vi "Actividad_01_Completa.vi"() -> ()   [LabVIEW 2025]
uses:
  <vilib>/Instr/_visa.llb/VISA Configure Serial Port (Instr).vi
panel:
  out "Contador":i32(knob) scale=-10000.0..10000.0
  out "Temperatura":dbl(slide) scale=0.0..100.0
  out "substring 2":string
  out "substring":string
  out "Temperatura buena":dbl
  out "Contador motor":i32
  in  "stop":bool
  in  "VISA resource name":refnum<visa-resource-name>
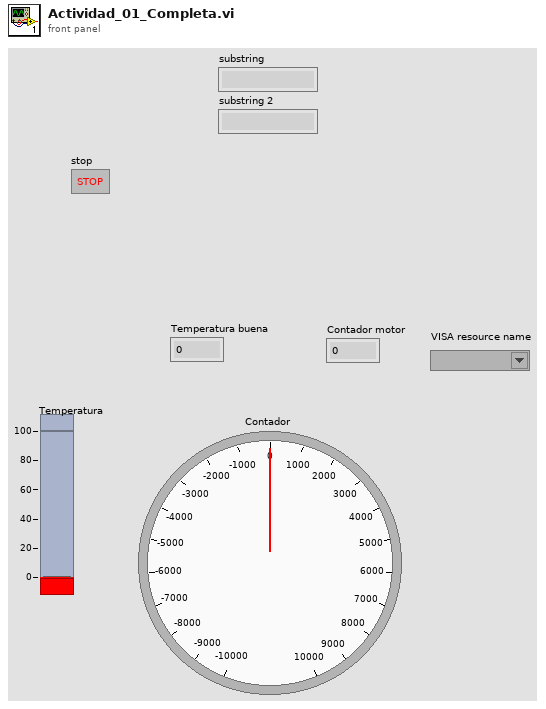
[diagram p1: front panel]
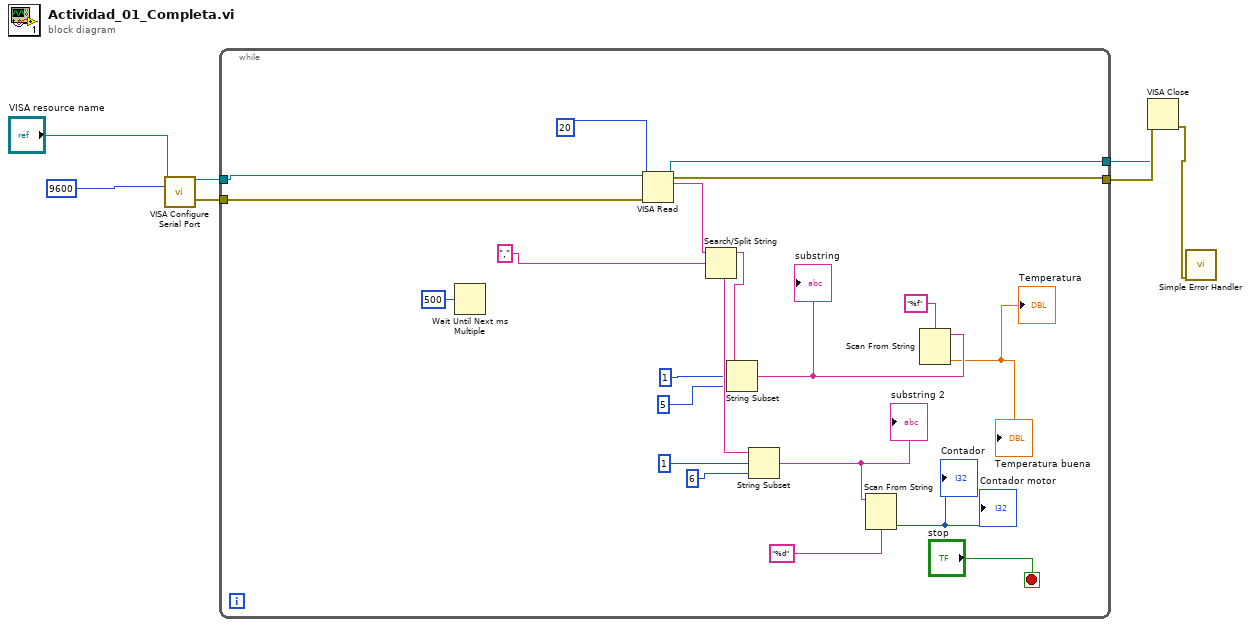
[diagram p0: block diagram]
diagram:
  n1 = call-poly "VISA Configure Serial Port"("VISA resource name"="VISA resource name", "baud rate (9600)"=u32 9600) -> ("VISA resource name out"=w5:refnum<visa-resource-name>, "error out"=w4:errorcluster)  [unwired: 12 in]
  n2 = while {
    tunnel: w5 -> [w10]
    tunnel: w4 -> [w11]
    tunnel: [w26] -> w3
    tunnel: [w25] -> w2
    stop <- "stop" stop-if-true
    n3 = Wait Until Next ms Multiple(millisecond multiple=u32 500) -> ()  [unwired: 1 out]
    n4 = VISA Read(VISA resource name=w10, byte count=u32 20, error in (no error)=w11) -> (VISA resource name out=w25:refnum<visa-resource-name>, read buffer=w12:string, error out=w26:errorcluster)  [unwired: 1 out]
    n5 = Search/Split String(string=w12, search string/char (-)=",") -> (substring before match=w14:string, match + rest of string=w19:string)  [unwired: 1 in, 1 out]
    n6 = String Subset(string=w14, offset (0)=1, length (rest)=5 ("length (rest)")) -> (substring=w18:string)
    "substring" <- w18
    n7 = String Subset(string=w19, offset (0)=1, length (rest)=6 ("length (rest)")) -> (substring=w21:string)
    "substring 2" <- w21
    n8 = Scan From String(format string="%d", input string=w21) -> (output 1=→"Contador motor" →"Contador":i32)  [unwired: 3 in, 3 out]
    n9 = Scan From String(format string="%f", input string=w18) -> (output 1=→"Temperatura buena" →"Temperatura":dbl)  [unwired: 3 in, 3 out]
  }
  n10 = VISA Close(VISA resource name=w2, error in (no error)=w3) -> (error out=w1:errorcluster)
  n11 = call <vilib>:"Simple Error Handler.vi"("error in (no error)"=w1) -> ()  [unwired: 4 in, 5 out]
